vi "Angles Get.vi"(8 "error in (no error)":errorcluster) -> (0 "error out":errorcluster, 2 "Angles (rad)":cluster{"theta":dbl, "phi":dbl, "psi":dbl} {"psi" format="%.1f"; "phi" format="%.1f"; "theta" format="%.1f"})   [LabVIEW 2017, in "Haptic Prog Interface.lvlib"]
doc: "Returns the 3 angles of the haptic pen in radians.\n\n<b>Angles:</b> Returns a cluster of the theta, phi, and psi angles of the pen (in units of radians)."
uses:
  Haptic Prog Interface.lvlib
  Haptic-Programming-Interface/src/x64/Debug/Haptic Programming Interface.dll
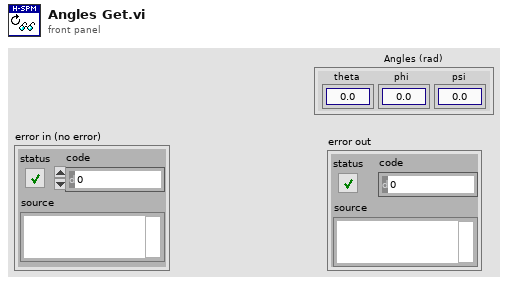
[diagram p1: front panel]
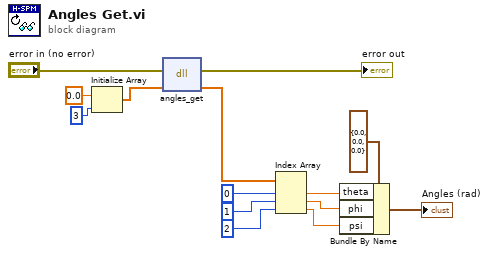
[diagram p0: block diagram]
diagram:
  n1 = Initialize Array(0.0 ("element"), 3 ("dimension size")) -> (w1:dbl[])
  n2 = dll-call lib="C:/Users/freem/Documents/GitHub/HapticSPM/Haptic-Programming-Interface/src/x64/Debug/Haptic Programming Interface.dll" fn="angles_get"(error in="error in (no error)", "output"=w1) -> (error out=→"error out":errorcluster, "output"=w12:dbl[])  [unwired: 3 in, 1 out]
  n3 = Index Array(array=w12, index #1=0 ("index"), index #2=1 ("index"), index #3=2 ("index")) -> (element #1=w8:dbl, element #2=w7:dbl, element #3=w6:dbl)
  n4 = Bundle By Name(cluster=cluster{"theta":dbl, "phi":dbl, "psi":dbl} {"theta"=0.0, "phi"=0.0, "psi"=0.0} ("Angles"), "theta"=w8, "phi"=w7, "psi"=w6) -> (→"Angles (rad)":cluster{"theta":dbl, "phi":dbl, "psi":dbl})
